vi "Agilent PSG MXG_Close.vi"(8 "error in":errorcluster {"code" format="%.0x"}, 11 "Handle":variant) -> (0 "error out":errorcluster {"code" format="%.0x"})   [LabVIEW 2015]
uses:
  <instrlib>/Agilent PSG MXG Series/Agilent PSG MXG Series.lvlib
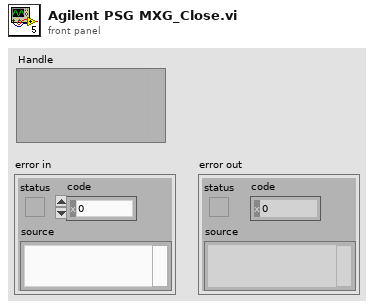
[diagram p1: front panel]
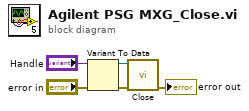
[diagram p0: block diagram]
diagram:
  n1 = Variant To Data(error in="error in", Variant="Handle") -> (data=w3:refnum<visa-resource-name>, error out=w1:errorcluster)  [unwired: 1 in]
  n2 = call <instrlib>:"Close.vi"("error in (no error)"=w1, "VISA resource name"=w3) -> ("error out"=→"error out":errorcluster)  [unwired: 9 in]
